vi "Aim2024.vi"() -> ()   [LabVIEW 2020]
uses:
  <vilib>/Utility/config.llb/Write Key (Double).vi
  <vilib>/Utility/config.llb/Write Key (I32).vi
  <vilib>/Utility/config.llb/Write Key (Boolean).vi
  <vilib>/Utility/config.llb/Write Key (String).vi
  <vilib>/Utility/config.llb/NI_LVConfig.lvlib
panel:
  in  "SAVE":bool
  out "当前时间":timestamp
  in  "外卖次数":enum16{"0次", "1次", "2次"}(ring)
  in  "体重":dbl
  in  "value":bool caption="房间干净么"
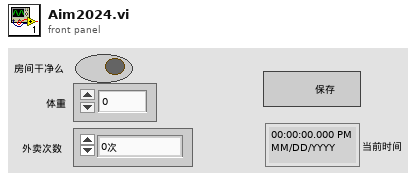
[diagram p1: front panel]
types:
  T1 = typedef "NI_LVConfig.lvlib/Config Data RefNum.ctl" = refnum<k1>
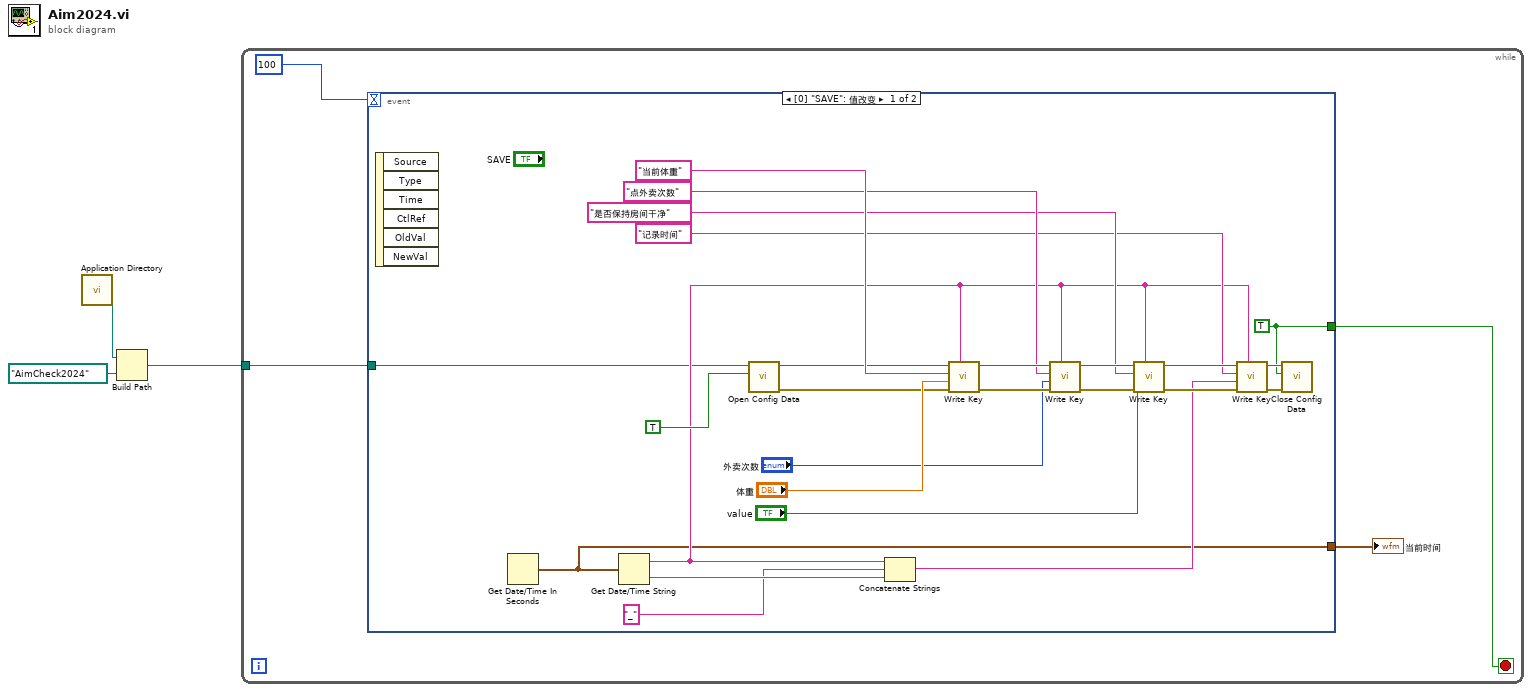
[diagram p0: block diagram]
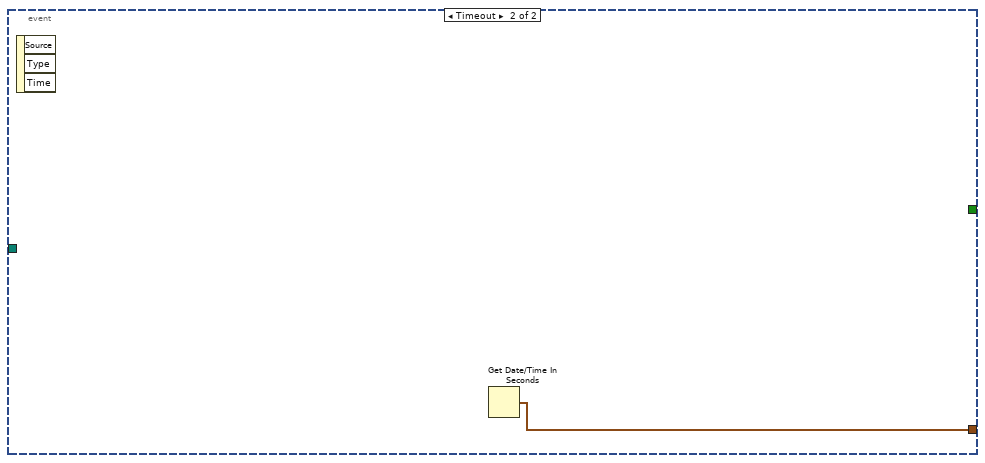
[diagram p2: hidden frame]
diagram:
  n1 = call <vilib>:"Application Directory.vi"() -> ("Application Directory"=w3:path)
  n2 = Build Path(base path=w3, name or relative path=path "AimCheck2024" ("名称或相对路径")) -> (appended path=w1:path)
  n3 = while {
    tunnel: w1 -> [w4]
    stop <- w7 stop-if-true
    n4 = event shown="[0] \"SAVE\": 值改变" {
      selector: _ -> [_ _]
      dyn-events: _ -> [_ _]
      timeout: 100 -> [_ _]
      tunnel: [w10 _] -> w7
      tunnel: [w9 w33] -> w6
      tunnel: w4 -> [w8 _]
      event "SAVE": Value Change {
        w10 = TRUE ("write file if changed (T)")
        n5 = event-data() -> ()  [unwired: 1 in, 6 out]
        n6 = Get Date/Time In Seconds() -> (seconds since 1Jan1904=w9:timestamp)
        n7 = Get Date/Time String(seconds (now)=w9) -> (date string=w14:string, time string=w25:string)  [unwired: 2 in]
        n8 = call <vilib>:"Open Config Data.vi"("create file if necessary (T)"=TRUE, "configuration file path"=w8) -> ("error out"=w11:errorcluster, "refnum"=w12:T1)  [unwired: 7 in, 1 out]
        n9 = Concatenate Strings(w14, "_" ("字符串"), w25) -> (w15:string)
        n10 = call-poly <vilib>:"Write Key.vi"("section"=w14, "error in (no error)"=w11, "value"="体重", "key"="当前体重", "refnum"=w12) -> ("error out"=w29:errorcluster, "refnum out"=w31:T1)  [unwired: 4 in, 1 out]
        n11 = call-poly <vilib>:"Write Key.vi"("section"=w14, "error in (no error)"=w29, "value"="外卖次数", "key"="点外卖次数", "refnum"=w31) -> ("error out"=w28:errorcluster, "refnum out"=w30:T1)  [unwired: 4 in, 1 out]
        n12 = call-poly <vilib>:"Write Key.vi"("section"=w14, "error in (no error)"=w28, "value"="value", "key"="是否保持房间干净", "refnum"=w30) -> ("error out"=w26:errorcluster, "refnum out"=w27:T1)  [unwired: 4 in, 1 out]
        n13 = call-poly <vilib>:"Write Key.vi"("section"=w14, "error in (no error)"=w26, "value"=w15, "key"="记录时间", "refnum"=w27) -> ("error out"=w21:errorcluster, "refnum out"=w22:T1)  [unwired: 4 in, 1 out]
        n14 = call <vilib>:"Close Config Data.vi"("error in (no error)"=w21, "write file if changed (T)"=w10, "refnum"=w22) -> ()  [unwired: 7 in, 2 out]
      }
      event Timeout {
        n15 = event-data() -> ()  [unwired: 1 in, 3 out]
        n16 = Get Date/Time In Seconds() -> (seconds since 1Jan1904=w33:timestamp)
      }
    }
    "当前时间" <- w6
  }
